vi "Main File - Kalibrasi MultiChannel Sensor - v05.vi"() -> ()   [LabVIEW 2018]
uses:
  <vilib>/Utility/error.llb/DialogType.ctl
  <vilib>/DAQmx/read.llb/DAQmx Read (Analog 1D Wfm NChan NSamp).vi
  <vilib>/Analysis/baseanly.llb/Mean (DBL).vi
  <vilib>/DAQmx/configure/timing.llb/DAQmx Timing (Sample Clock).vi
  <vilib>/DAQmx/miscellaneous.llb/DAQmx Fill In Error Info.vi
  <resource>/objmgr/daqmx.rc
  <vilib>/Analysis/NI_AALBase.lvlib
  <vilib>/Analysis/NI_AALPro.lvlib
panel:
  in  "Kalibrasi":T1(ring)
  in  "Default":bool=TRUE
  in  "Input Kalibrasi":dbl min=-22.0 max=22.0
  in  "Max Input":dbl=22.0
  in  "Min Input":dbl=-22.0
  out "Iterasi":i32
  out "Stabil Log OK":bool
  out "Stabil Log data":i32
  in  "Calibration Action":enum32{"To Excel", "Waiting", "Stabil Log"}(radio)=enum."Waiting"
  out "Mode":string
  in  "Main LogFile Path":path=path "F:/Kerjaan Kantor/2023/LabView Kalibrasi/LabVIEW .vi File Final/Multiple Channel Sensor/LogData/tes-5ch-02.txt" caption="Filename"
  in  "Tab Control":T2(tab)
  out "Chart Stabil Log":waveform(dbl)[](graph)
  out "Waveform Chart Non Stop":waveform(dbl)[](graph)
  out "Indikator Input Kalibrasi":dbl(slide) min=-22.0 max=22.0 scale=-22.0..22.0
  out "Export To Excel":bool
  in  "Excel Path":path=path "F:/Kerjaan Kantor/2023/LabView Kalibrasi/LabVIEW .vi File Final/Multiple Channel Sensor/AnalisaData/Template Analisa Kalibrasi WHS P.1-5 -22cm to 22cm mmyyyy .xlsx"
  out "Tabel Mean Zero":dbl[][](array[numeric]) format="%#_4g"
  out "Data Kalibrasi":dbl(slide) min=-22.0 max=22.0 scale=-22.0..22.0
  in  "Pilih Sensor":i32=1 min=1 max=5 step=1
  out "R-square":dbl format="%#_3g"
  out "Slope":dbl format="%#_4g"
  out "Intercept":dbl format="%#_4g"
  out "Sensor":cluster{dbl[], dbl[]}(graph)
  out "Tabel Slope, Intercept dan R Square":dbl[][](array[numeric]) format="%#_4g"
  in  "DAQ Channel":refnum<k21>="Simulated_AI_Ch0:4"
  in  "stop":bool
  # "Data\nKalibrasi"
  # "S 3"
  # "S 4"
  # "S 1"
  # "S 2"
  # "S 5"
  # "R Square"
  # "Sensor No"
  # "Slope"
  # "Intercept"
  # "Note \nTo export this tabel:\n1. Click this table to select all of this table content.\n2.  Right click this table then choose export to clipboard or to excel"
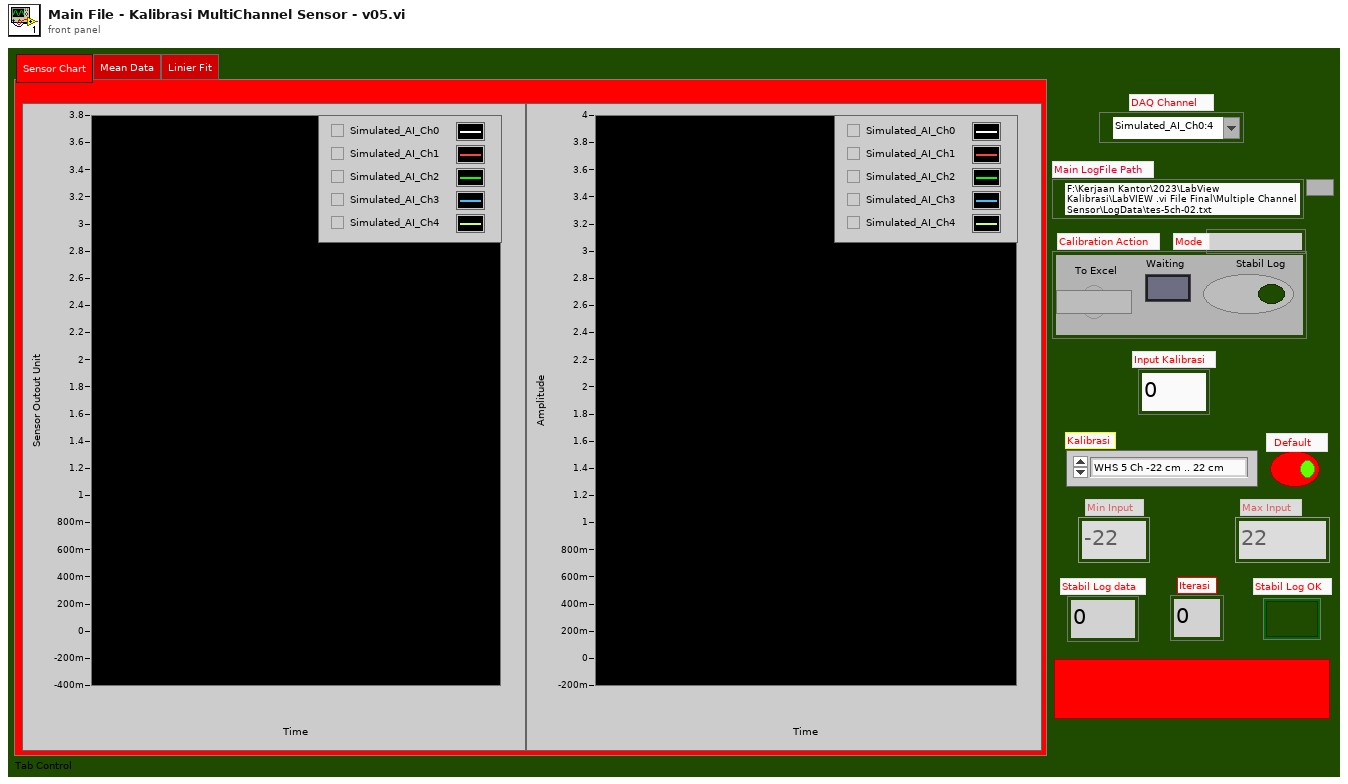
[diagram p1: front panel]
types:
  T1 = enum16{"WHS 5 Ch -22 cm .. 22 cm", "WHS 5 Ch -20 cm .. 20 cm", "WHS 1 Ch -20 cm .. 20 cm", "R-56 Resistance", "H-39 Open Water Thrust", "H-39 Open Water Torsi CW", "H-39 Open Water Torsi CCW", "R-31 Self Propulsi Thrust", "R-31 Self Propulsi Torsi CW", "R-31 Self Propulsi Torsi CCW", "R-33 Self Propulsi Thrust", "R-33 Self Propulsi Torsi CW", "R-33 Self Propulsi CCW", "Other Sensor Data"}
  T2 = enum32{"Sensor Chart", "Mean Data", "Linier Fit"}
  T3 = typedef "DialogType.ctl" = u16
  T4 = enum8{"Enabled", "Disabled", "Disabled and Grayed Out"}
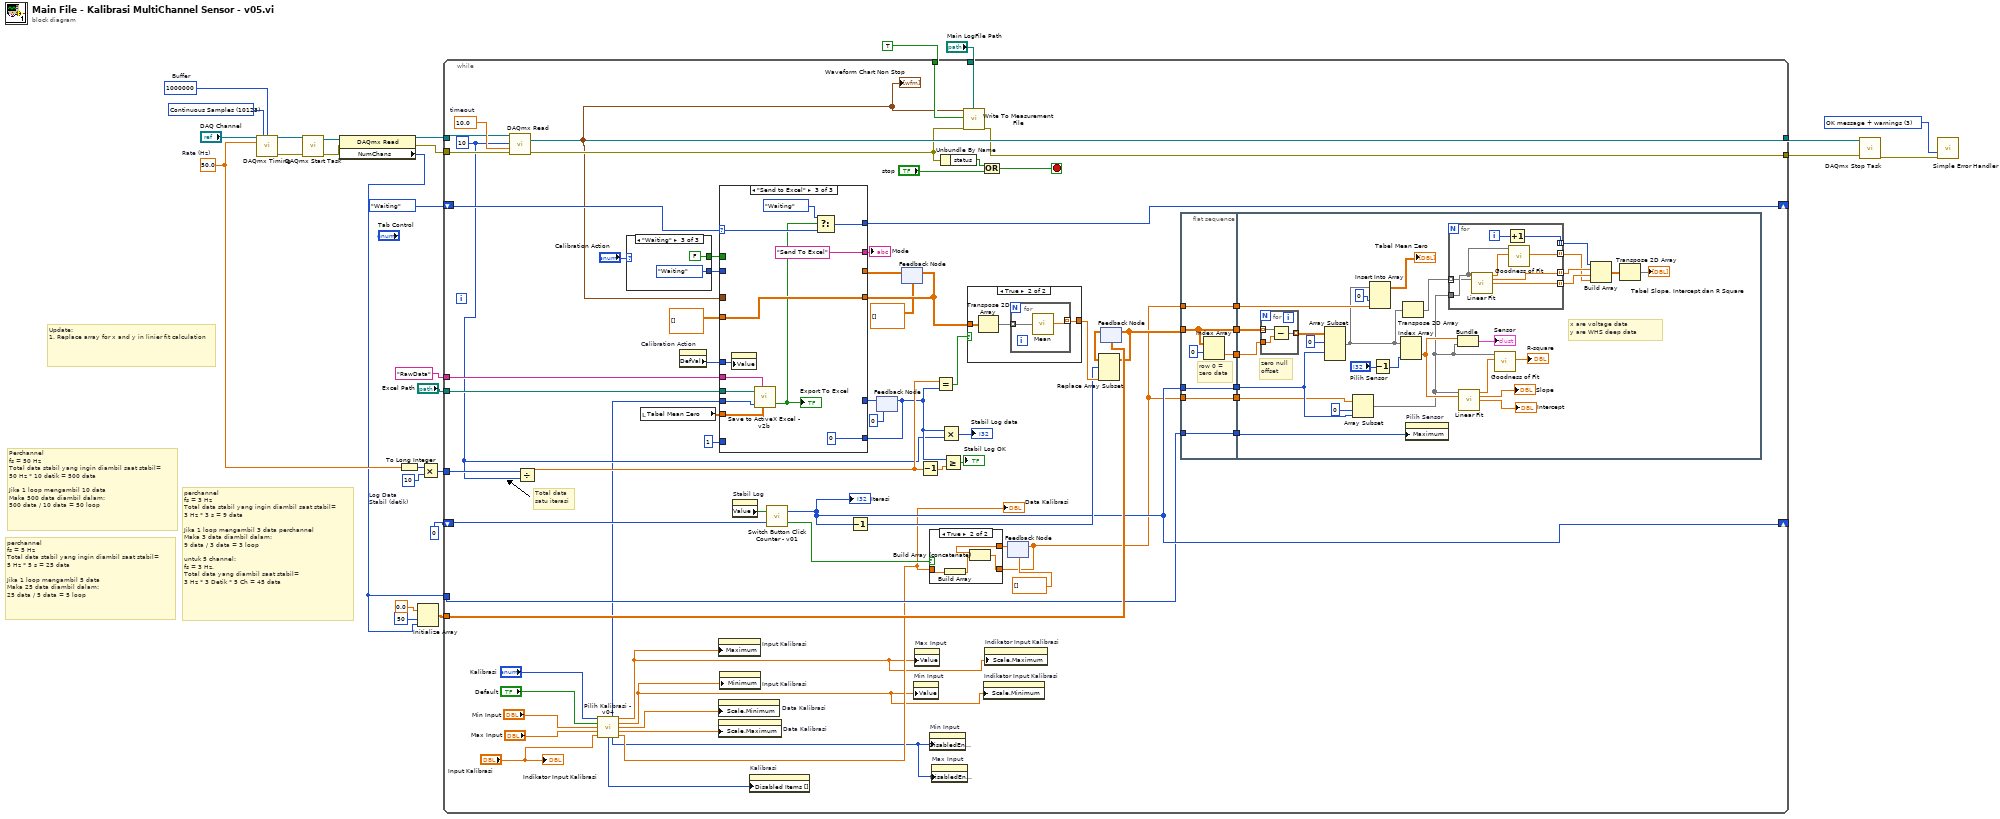
[diagram p0: block diagram]
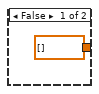
[diagram p3: hidden frame]
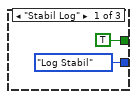
[diagram p4: hidden frame]
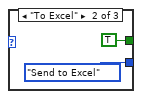
[diagram p5: hidden frame]
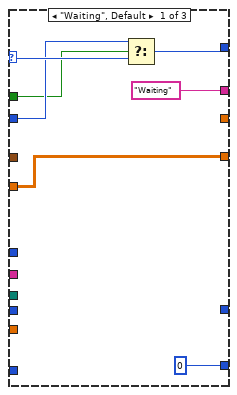
[diagram p6: hidden frame]
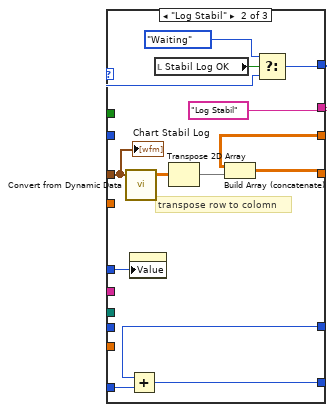
[diagram p7: hidden frame]
diagram:
  w8 = 50.0  # Rate (Hz)
  w9 = 1000000  # Buffer
  w10 = 10123 items=["Finite Samples"=10178, "Continuous Samples"=10123, "Hardware Timed Single Point"=12522] ("Sample Mode")
  w11 = 10  # Log Data Stabil (detik)
  w20 = T3 3 items=["no dialog", "OK message", "continue or stop message", "OK message + warnings", "continue/stop + warnings"] ("type of dialog (OK msg:1)")
  # "Update:\n1. Replace array for x and y in linier fit calculation"
  # "perchannel \nfs = 3 Hz\nTotal data stabil yang ingin diambil saat stabil=\n3 Hz * 3 s = 9 data\n\nJika 1 loop mengambil 3 data perchannel\nMaka 3 data diambil dalam:\n9 data / 3 data = 3 loop \n\nuntuk 5 channel:\nfs = 3 Hz.\nTotal data yang diambil saat stabil=\n3 Hz * 3 Detik * 5 Ch = 45 data"
  # "perchannel \nfs = 5 Hz\nTotal data stabil yang ingin diambil saat stabil=\n5 Hz * 5 s = 25 data\n\nJika 1 loop mengambil 5 data\nMaka 25 data diambil dalam:\n25 data / 5 data = 5 loop"
  # "Perchannel\nfs = 50 Hz\nTotal data stabil yang ingin diambil saat stabil=\n50 Hz * 10 detik = 500 data\n\nJika 1 loop mengambil 10 data\nMaka 500 data diambil dalam:\n500 data / 10 data = 50 loop"
  n1 = call-poly <vilib>:"DAQmx Timing.vi"("task/channels in"="DAQ Channel", "sample mode"=w10, "samples per channel"=w9, "rate"=w8) -> ("task out"=w27:refnum<k21>, "error out"=w26:errorcluster)  [unwired: 10 in]
  n2 = call <vilib>:"DAQmx Start Task.vi"("task/channels in"=w27, "error in"=w26) -> ("task out"=w5:refnum<k21>, "error out"=w4:errorcluster)  [unwired: 12 in]
  n3 = property class="DAQmx Read"(reference=w5, error in=w4) -> (reference out=w2:refnum<k21>, error out=w3:errorcluster, "NumChans"=w1:u32)
  n4 = To Long Integer(number=w8) -> (32bit integer=w15:i32)
  n5 = Initialize Array(0.0 ("element"), 50 ("dimension size"), w1) -> (w16:dbl[][])
  n6 = Multiply(x=w15, y=w11) -> (x*y=w14:i32)
  n7 = while {
    tunnel: w3 -> [w95]
    tunnel: w2 -> [w94]
    tunnel: [w89] -> w24
    tunnel: [w91] -> w23
    tunnel: "Main LogFile Path" -> [w88]
    tunnel: TRUE ("Enable\nRekam") -> [w87]
    shift-right: [w85] -> _
    shift-left: enum16{"Waiting", "Log Stabil", "Send to Excel"}."Waiting" -> [w83]
    tunnel: w16 -> [w64]
    tunnel: w14 -> [w68]
    shift-right: [w53] -> _
    shift-left: 0 ("Numeric") -> [w77]
    tunnel: "Excel Path" -> [w75]
    tunnel: "RawData" ("Excel Sheet") -> [w74]
    tunnel: w1 -> [w48]
    stop <- w86 stop-if-true
    w50 = 10 ("number of samples per channel")
    w96 = 10.0  # timeout
    # "Total data \nsatu iterasi"
    n8 = call-poly <vilib>:"DAQmx Read.vi"("task/channels in"=w94, "number of samples per channel"=w50, "timeout"=w96, "error in"=w95) -> ("task out"=w91:refnum<k21>, "data"=w79:waveform(dbl)[], "error out"=w90:errorcluster)  [unwired: 9 in]
    "Waveform Chart Non Stop" <- w79
    n9 = Divide(x=w68, y=w50) -> (x/y=w60:dbl)
    n10 = call "Pilih Kalibrasi - v04.vi"("Kalibrasi"="Kalibrasi", "Default"="Default", "Min In"="Min Input", "Max In"="Max Input", "Input"="Input Kalibrasi") -> ("Ind.Col"=w40:i32, "Max Input"=w32:dbl, "Min Input"=w31:dbl, "Min Data Kalibrasi"=w33:dbl, "Max Data Kalibrasi"=w34:dbl, "Disabled Items []"=w28:i32[], "MaxMinEnabled"=w30:T4, "Data Kalibrasi"=w35:dbl)  [unwired: 3 in]
    "Data Kalibrasi" <- w35
    n11 = case shown="\"Waiting\"" "Calibration Action" {
      tunnel: [enum16{"Waiting", "Log Stabil", "Send to Excel"}."Log Stabil" enum16{"Waiting", "Log Stabil", "Send to Excel"}."Send to Excel" enum16{"Waiting", "Log Stabil", "Send to Excel"}."Waiting"] -> w81
      tunnel: [TRUE TRUE FALSE] -> w80
      frame "Stabil Log" {
      }
      frame "To Excel" {
      }
      frame "Waiting" {
      }
    }
    n12 = local read "Tabel Mean Zero"() -> (w58:dbl[][])
    n13 = property on="Calibration Action" class="RadioBtnsControl (strict)"() -> ("DefVal"=w70:enum32{"To Excel", "Waiting", "Stabil Log"})  [unwired: 2 in, 2 out]
    n14 = property on="Input Kalibrasi" class="DigNum (strict)"("Maximum"=w32) -> ()  [unwired: 2 in, 2 out]
    n15 = property on="Data Kalibrasi" class="Slide (strict)"("Scale.Minimum"=w33) -> ()  [unwired: 2 in, 2 out]
    n16 = property on="Data Kalibrasi" class="Slide (strict)"("Scale.Maximum"=w34) -> ()  [unwired: 2 in, 2 out]
    n17 = property on="Input Kalibrasi" class="DigNum (strict)"("Minimum"=w31) -> ()  [unwired: 2 in, 2 out]
    n18 = property on="Stabil Log" class="Bool (strict)"() -> ("Value"=w76:bool)  [unwired: 2 in, 2 out]
    n19 = property on="Kalibrasi" class="Enum (strict)"("Disabled Items []"=w28) -> ()  [unwired: 2 in, 2 out]
    n20 = call "Switch Button Click Counter - v01.vi"("Numeric"=w77, "Klik"=w76) -> ("Output"=w45:bool, "Klik Counter"=w53:i32)
    "Iterasi" <- w53
    n21 = Decrement(x=w53) -> (x-1=w55:i32)
    n22 = feedback #1(0) -> (w71:i32)
    n23 = feedback #2(dbl[][] []) -> (w66:dbl[][])
    n24 = case shown="\"Send to Excel\"" w83 {
      selector: w83 -> [w164 w177 w189]
      tunnel: [w166 w178 w191] -> w85
      tunnel: ["Waiting" "Log Stabil" "Send To Excel"] -> w84
      tunnel: w81 -> [w163 _ _]
      tunnel: w80 -> [w162 _ _]
      tunnel: w79 -> [_ w167 _]
      tunnel: w58 -> [_ _ w182]
      tunnel: w75 -> [_ _ w188]
      tunnel: w74 -> [_ _ w184]
      tunnel: 1 -> [_ w175 _]
      tunnel: [0 w174 0] -> w51
      tunnel: w71 -> [_ w173 _]
      tunnel: w70 -> [_ w172 w186]
      tunnel: [w160 w169 w185] -> w65
      tunnel: dbl[][] [] -> [w160 _ w185]
      tunnel: w66 -> [_ w170 _]
      tunnel: w40 -> [_ _ w181]
      frame "Waiting", Default {
        n25 = Select(t=w163, s=w162, f=w164) -> (s? t:f=w166:enum16{"Waiting", "Log Stabil", "Send to Excel"})
      }
      frame "Log Stabil" {
        # "transpose row to colomn"
        n26 = call "Convert from Dynamic Data"("Dynamic Data Type"=w167) -> ("Array"=w171:dbl[][])  [unwired: 3 in]
        n27 = Add(x=w173, y=w175) -> (x+y=w174:i32)
        n28 = property on="Calibration Action" class="RadioBtnsControl (strict)"("Value"=w172) -> ()  [unwired: 2 in, 2 out]
        n29 = local read "Stabil Log OK"() -> (w176:bool)
        n30 = Transpose 2D Array(2D array=w171) -> (transposed array=w168:dbl[][])
        n31 = Build Array (concatenate)(w170, w168) -> (w169:dbl[][])
        n32 = Select(t=enum16{"Waiting", "Log Stabil", "Send to Excel"}."Waiting", s=w176, f=w177) -> (s? t:f=w178:enum16{"Waiting", "Log Stabil", "Send to Excel"})
        "Chart Stabil Log" <- w167
      }
      frame "Send to Excel" {
        n33 = property on="Calibration Action" class="RadioBtnsControl (strict)"("Value"=w186) -> ()  [unwired: 2 in, 2 out]
        n34 = call "Save to ActiveX Excel - v2b.vi"("Path"=w188, "Excel._SheetName"=w184, "Ikol"=w181, "Table Mean Data"=w182) -> ("OK"=w183:bool)  [unwired: 1 in, 1 out]
        "Export To Excel" <- w183
        n35 = Select(t=enum16{"Waiting", "Log Stabil", "Send to Excel"}."Waiting", s=w183, f=w189) -> (s? t:f=w191:enum16{"Waiting", "Log Stabil", "Send to Excel"})
      }
    }
    "Mode" <- w84
    n36 = feedback-in #1(w51) -> ()
    n37 = feedback-in #2(w65) -> ()
    n38 = property on="Min Input" class="DigNum (strict)"("Value"=w31) -> ()  [unwired: 2 in, 2 out]
    n39 = property on="Max Input" class="DigNum (strict)"("Value"=w32) -> ()  [unwired: 2 in, 2 out]
    n40 = Decrement(x=w60) -> (x-1=w69:dbl)
    n41 = property on="Min Input" class="DigNum (strict)"("DisabledEnum"=w30) -> ()  [unwired: 2 in, 2 out]
    n42 = property on="Max Input" class="DigNum (strict)"("DisabledEnum"=w30) -> ()  [unwired: 2 in, 2 out]
    n43 = Equal?(x=w60, y=w51) -> (x = y?=w61:bool)
    n44 = Unbundle By Name(w90) -> ("status"=w93:bool)
    n45 = Multiply(x=w51, y=w50) -> (x*y=→"Stabil Log data":i32)
    n46 = Greater Or Equal?(x=w51, y=w69) -> (x >= y?=→"Stabil Log OK":bool)
    n47 = call "Write To Measurement File"("Signals"=w79, "Enable"=w87, "error in (no error)"=w90, "Filename"=w88) -> ("error out"=w89:errorcluster)  [unwired: 13 in, 2 out]
    n48 = case shown="True" w61 {
      tunnel: w65 -> [_ w151]
      tunnel: [dbl[] [] w149] -> w62
      frame False {
      }
      frame True {
        n49 = Transpose 2D Array(2D array=w151) -> (transposed array=w150:dbl[][])
        n50 = for {
          tunnel: w150 -> [w153] mode=indexing
          tunnel: [w152] -> w149 mode=indexing
          n51 = call-poly <vilib>:"Mean.vi"("X"=w153) -> ("mean"=w152:dbl)  [unwired: 1 out]
        }
      }
    }
    n52 = property on="Indikator Input Kalibrasi" class="Slide (strict)"("Scale.Minimum"=w31) -> ()  [unwired: 2 in, 2 out]
    n53 = Compound Arithmetic op=OR(w93, "stop") -> (w86:bool)
    n54 = property on="Indikator Input Kalibrasi" class="Slide (strict)"("Scale.Maximum"=w32) -> ()  [unwired: 2 in, 2 out]
    n55 = feedback #3(dbl[] []) -> (w46:dbl[])
    n56 = case shown="True" w45 {
      tunnel: w35 -> [_ w101]
      tunnel: [w97 w99] -> w41
      tunnel: w46 -> [w97 w98]
      frame False {
      }
      frame True {
        n57 = Build Array(w101) -> (w100:dbl[])
        n58 = Build Array (concatenate)(w98, w100) -> (w99:dbl[])
      }
    }
    n59 = feedback-in #3(w41) -> ()
    n60 = feedback #4(w64) -> (w63:dbl[][])
    n61 = Replace Array Subset(array=w63, new element=w62, index (row)=w55) -> (w44:dbl[][])  [unwired: 1 in]
    n62 = feedback-in #4(w44) -> ()
    n63 = flat-sequence {
      tunnel: w44 -> [w107]
      tunnel: [w107] -> w57
      tunnel: [w106] -> w56
      tunnel: w53 -> [w105]
      tunnel: [w105] -> w54
      tunnel: [w104] -> w49
      tunnel: w48 -> [w104]
      tunnel: [w103] -> w43
      tunnel: w41 -> [w103]
      tunnel: w41 -> [w102]
      tunnel: [w102] -> w42
      tunnel: w57 -> [w136]
      tunnel: w56 -> [w135]
      tunnel: w54 -> [w131]
      tunnel: w49 -> [w126]
      tunnel: w43 -> [w125]
      tunnel: w42 -> [w124]
      frame #0 {
        # "row 0 =\nzero data"
        n64 = Index Array(array=w107, index (row)=0) -> (element=w106:dbl[])  [unwired: 1 in]
      }
      frame #1 {
        # "x are voltage data\ny are WHS deep data"
        # "zero null\noffset"
        n65 = for {
          tunnel: w136 -> [w147] mode=indexing
          tunnel: w135 -> [w146]
          tunnel: [w145] -> w133 mode=indexing
          n66 = Subtract(x=w147, y=w146) -> (x-y=w145:dbl[])
        }
        n67 = Array Subset(array=w133, index (row)=0 ("index"), length (row)=w131) -> (w118:dbl[][])  [unwired: 2 in]
        n68 = Array Subset(array=w125, index=0, length=w131) -> (w109:dbl[])
        n69 = Insert Into Array(array=w118, index (col)=0 ("disabled index (col)"), new element=w124) -> (→"Tabel Mean Zero":dbl[][])  [unwired: 1 in]
        n70 = Decrement(x="Pilih Sensor") -> (x-1=w127:i32)
        n71 = Index Array(array=w118, index (col)=w127) -> (element=w110:dbl[])  [unwired: 1 in]
        n72 = Transpose 2D Array(2D array=w118) -> (transposed array=w117:dbl[][])
        n73 = property on="Pilih Sensor" class="DigNum (strict)"("Maximum"=w126) -> ()  [unwired: 2 in, 2 out]
        n74 = for {
          tunnel: w109 -> [w138]
          tunnel: [w143] -> w114 mode=indexing
          tunnel: [w142] -> w116 mode=indexing
          tunnel: [w141] -> w115 mode=indexing
          tunnel: w117 -> [w137] mode=indexing
          tunnel: [w139] -> w111 mode=indexing
          i -> [w140]
          n75 = call <vilib>:"Linear Fit.vi"("Y"=w138, "X"=w137) -> ("Best Linear Fit"=w144:dbl[], "slope"=w142:dbl, "intercept"=w141:dbl)  [unwired: 9 in, 2 out]
          n76 = Increment(x=w140) -> (x+1=w139:i32)
          n77 = call <vilib>:"Goodness of Fit.vi"("Best Fit"=w144, "Y"=w138) -> ("R-square"=w143:dbl)  [unwired: 6 in, 3 out]
        }
        n78 = Bundle(w110, w109) -> (→"Sensor":cluster{dbl[], dbl[]})  [unwired: 1 in]
        n79 = call <vilib>:"Linear Fit.vi"("Y"=w109, "X"=w110) -> ("Best Linear Fit"=w130:dbl[], "slope"=→"Slope":dbl, "intercept"=→"Intercept":dbl)  [unwired: 9 in, 2 out]
        n80 = call <vilib>:"Goodness of Fit.vi"("Best Fit"=w130, "Y"=w109) -> ("R-square"=→"R-square":dbl)  [unwired: 6 in, 3 out]
        n81 = Build Array(w111, w116, w115, w114) -> (w113:dbl[][])
        n82 = Transpose 2D Array(2D array=w113) -> (transposed array=→"Tabel Slope, Intercept dan R Square":dbl[][])
      }
    }
    "Indikator Input Kalibrasi" <- "Input Kalibrasi"
  }
  n83 = call <vilib>:"DAQmx Stop Task.vi"("task/channels in"=w23, "error in"=w24) -> ("error out"=w25:errorcluster)  [unwired: 12 in, 1 out]
  n84 = call <vilib>:"Simple Error Handler.vi"("type of dialog (OK msg:1)"=w20, "error in (no error)"=w25) -> ()  [unwired: 3 in, 5 out]
